vi "QueuedWriteToDatabase.vi"(8 "error in":errorcluster, 10 "Stop Flag Reference":refnum<vi>, 11 "queue":refnum<queue>) -> (0 "error out":errorcluster)   [LabVIEW 2014]
uses:
  <vilib>/addons/database/Connection.llb/Conn ObjectReference.ctl
  <vilib>/addons/database/NI_Database_API.lvlib
panel:
  out "Database Writing Source":i32
  out "Database Table":string
  out "Database Writing Error":bool
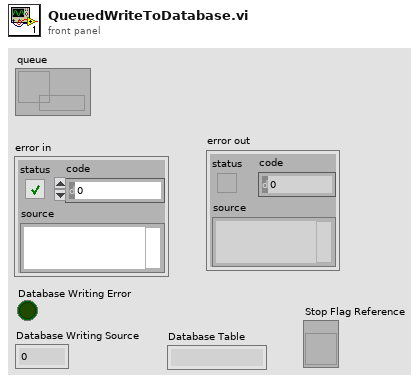
[diagram p1: front panel]
types:
  T1 = cluster{"setup":u8, "session_start_time":u64, "stim_start_time":u64, "time":u64}
  T2 = cluster{"setup":u8, "subject_id":i32, "session_start_time":dbl, "stim_start_time":dbl, "stim_path":path, "exp_type":string}
  T3 = cluster{"setup":u8, "subject_id":i32, "session_start_time":dbl, "stim_start_time":dbl, "time":dbl}
  T4 = cluster{"setup":u8, "subject_id":i32, "session_start_time":dbl, "stim_start_time":dbl, "beh_start_time":dbl, "beh_path":path, "beh_traces_type":string, "beh_stop_time":dbl}
  T5 = cluster{"setup":u8, "subject_id":i32, "session_start_time":dbl, "ephys_start_time":dbl, "ephys_path":path, "ephys_task":string, "ephys_stop_time":dbl}
  T6 = cluster{"setup":u8, "subject_id":u64, "session_start_time":dbl, "channel":u64, "counter":u64, "time":u64}
  T7 = cluster{"setup":u8, "subject_id":i32, "experimenter":string, "session_start_time":dbl, "session_path":path, "session_datetime":timestamp, "session_stop_time":dbl}
  T8 = cluster{"setup":u8, "subject_id":i32, "session_start_time":dbl, "stim_start_time":dbl, "stim_path":path, "exp_type":string, "stim_stop_time":dbl}
  T9 = typedef "NI_Database_API.lvlib/Conn ObjectReference.ctl" = refnum<k1>
  T10 = cluster{cluster{"reference":T9, "table":string, "columns":string[], i32}, "Variant":variant}
  T11 = cluster{"reference":T9, "table":string, "columns":string[], i32}
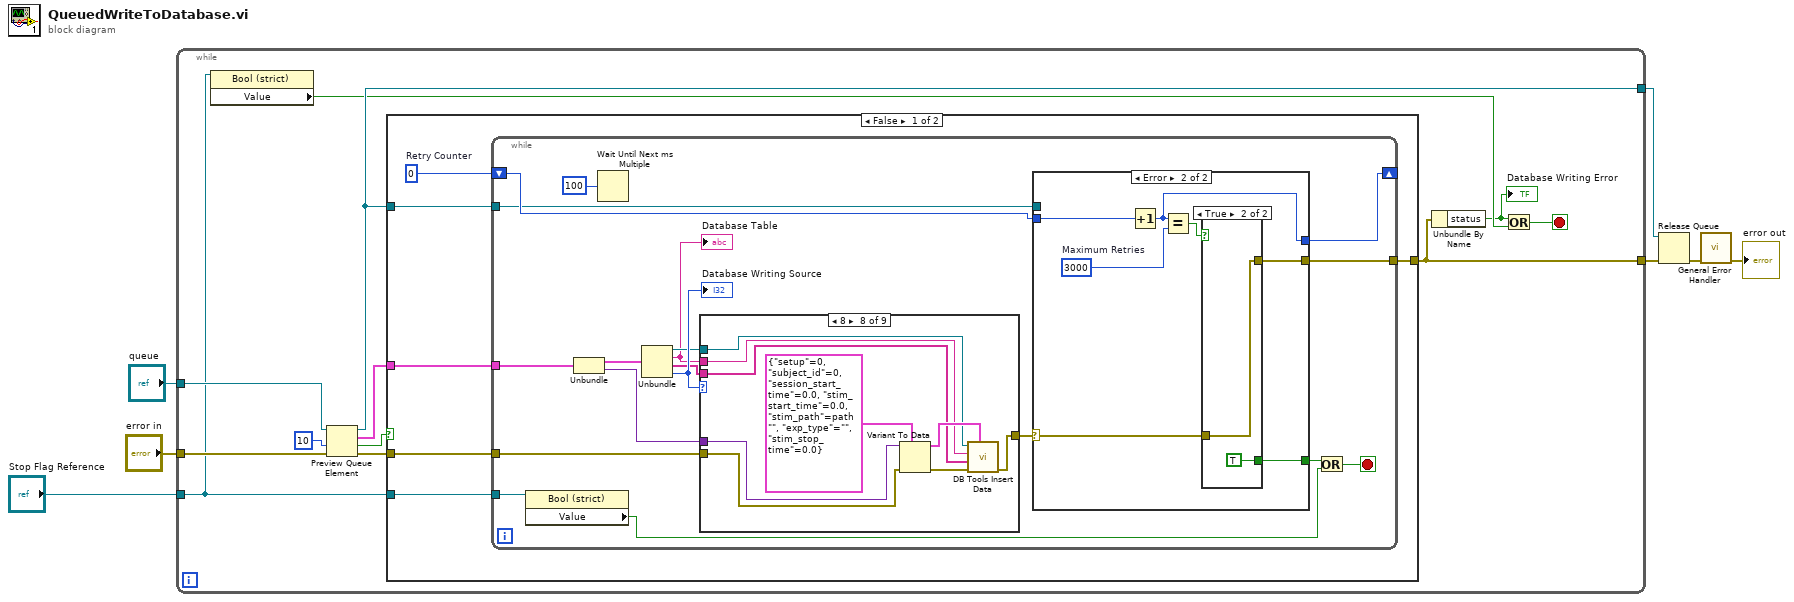
[diagram p0: block diagram]
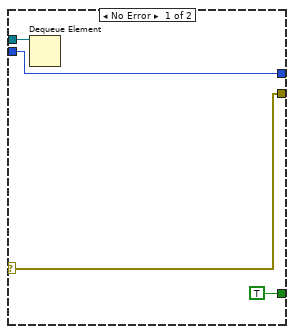
[diagram p2: hidden frame]
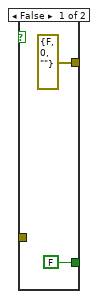
[diagram p3: hidden frame]
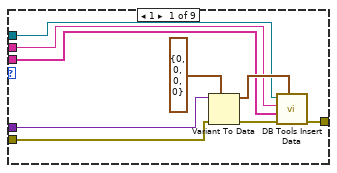
[diagram p4: hidden frame]
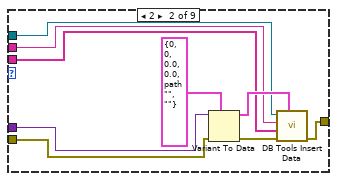
[diagram p5: hidden frame]
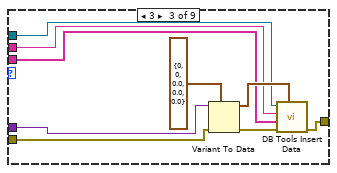
[diagram p6: hidden frame]
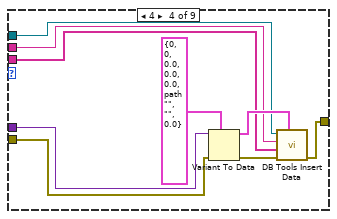
[diagram p7: hidden frame]
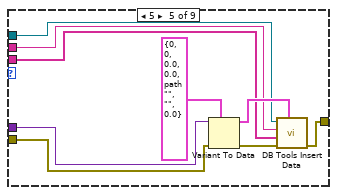
[diagram p8: hidden frame]
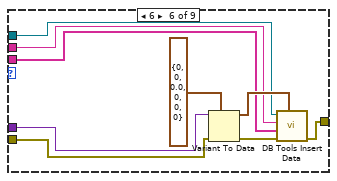
[diagram p9: hidden frame]
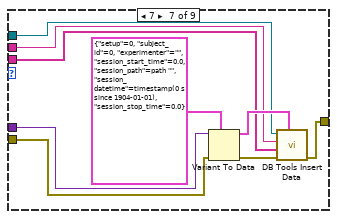
[diagram p10: hidden frame]
diagram:
  n1 = while {
    tunnel: "error in" -> [w13]
    tunnel: [w11] -> w4
    tunnel: [w12] -> w3
    tunnel: "Stop Flag Reference" -> [w8]
    tunnel: "queue" -> [w14]
    stop <- w16 stop-if-true
    n2 = property class="Bool (strict)"(reference=w8) -> ("Value"=w10:bool)  [unwired: 1 in, 2 out]
    n3 = Preview Queue Element(queue=w14, timeout in ms (-1)=10, error in (no error)=w13) -> (queue out=w11:refnum<queue>, element=w15:T10, timed out?=w18:bool, error out=w17:errorcluster)
    n4 = case shown="False" w18 {
      tunnel: w15 -> [w25 _]
      tunnel: w17 -> [w24 w132]
      tunnel: [w22 w132] -> w12
      tunnel: w11 -> [w21 _]
      tunnel: w8 -> [w20 _]
      frame False {
        w23 = 0  # Retry Counter
        n5 = while {
          tunnel: w25 -> [w43]
          tunnel: w24 -> [w39]
          shift-right: [w31] -> _
          shift-left: w23 -> [w33]
          tunnel: [w32] -> w22
          tunnel: w21 -> [w30]
          tunnel: w20 -> [w29]
          stop <- w27 stop-if-true
          n6 = property class="Bool (strict)"(reference=w29) -> ("Value"=w26:bool)  [unwired: 1 in, 2 out]
          n7 = Unbundle(w43) -> (w42:T11, "Variant"=w41:variant)
          n8 = Wait Until Next ms Multiple(millisecond multiple=u32 100) -> ()  [unwired: 1 out]
          n9 = Unbundle(w42) -> ("reference"=w38:T9, "table"=w37:string, "columns"=w36:string[], w40:i32)
          "Database Writing Source" <- w40
          "Database Table" <- w37
          n10 = case shown="8" w40 {
            tunnel: w41 -> [w67 w75 w84 w87 w98 w105 w116 w124 _]
            tunnel: w39 -> [w65 w74 w83 w88 w97 w107 w115 w125 w131]
            tunnel: [w59 w68 w77 w89 w96 w106 w114 w123 w131] -> w34
            tunnel: w38 -> [w63 w72 w81 w90 w99 w108 w119 w128 _]
            tunnel: w37 -> [w62 w71 w80 w91 w100 w109 w118 w127 _]
            tunnel: w36 -> [w61 w70 w79 w92 w101 w110 w117 w126 _]
            frame 1 {
              n11 = Variant To Data(error in=w65, type=T1 {"setup"=0, "session_start_time"=0, "stim_start_time"=0, "time"=0} ("output cluster"), Variant=w67) -> (data=w64:T1, error out=w60:errorcluster)
              n12 = call <vilib>:"DB Tools Insert Data.vi"("data"=w64, "error in (no error)"=w60, "columns"=w61, "table"=w62, "connection reference"=w63) -> ("error out"=w59:errorcluster)  [unwired: 5 in, 1 out]
            }
            frame 2 {
              n13 = Variant To Data(error in=w74, type=T2 {"setup"=0, "subject_id"=0, "session_start_time"=0.0, "stim_start_time"=0.0, "stim_path"=path "", "exp_type"=""} ("output cluster"), Variant=w75) -> (data=w73:T2, error out=w69:errorcluster)
              n14 = call <vilib>:"DB Tools Insert Data.vi"("data"=w73, "error in (no error)"=w69, "columns"=w70, "table"=w71, "connection reference"=w72) -> ("error out"=w68:errorcluster)  [unwired: 5 in, 1 out]
            }
            frame 3 {
              n15 = Variant To Data(error in=w83, type=T3 {"setup"=0, "subject_id"=0, "session_start_time"=0.0, "stim_start_time"=0.0, "time"=0.0} ("output cluster"), Variant=w84) -> (data=w82:T3, error out=w78:errorcluster)
              n16 = call <vilib>:"DB Tools Insert Data.vi"("data"=w82, "error in (no error)"=w78, "columns"=w79, "table"=w80, "connection reference"=w81) -> ("error out"=w77:errorcluster)  [unwired: 5 in, 1 out]
            }
            frame 4 {
              n17 = Variant To Data(error in=w88, type=T4 {"setup"=0, "subject_id"=0, "session_start_time"=0.0, "stim_start_time"=0.0, "beh_start_time"=0.0, "beh_path"=path "", "beh_traces_type"="", "beh_stop_time"=0.0} ("output cluster"), Variant=w87) -> (data=w93:T4, error out=w94:errorcluster)
              n18 = call <vilib>:"DB Tools Insert Data.vi"("data"=w93, "error in (no error)"=w94, "columns"=w92, "table"=w91, "connection reference"=w90) -> ("error out"=w89:errorcluster)  [unwired: 5 in, 1 out]
            }
            frame 5 {
              n19 = Variant To Data(error in=w97, type=T5 {"setup"=0, "subject_id"=0, "session_start_time"=0.0, "ephys_start_time"=0.0, "ephys_path"=path "", "ephys_task"="", "ephys_stop_time"=0.0} ("output cluster"), Variant=w98) -> (data=w102:T5, error out=w103:errorcluster)
              n20 = call <vilib>:"DB Tools Insert Data.vi"("data"=w102, "error in (no error)"=w103, "columns"=w101, "table"=w100, "connection reference"=w99) -> ("error out"=w96:errorcluster)  [unwired: 5 in, 1 out]
            }
            frame 6 {
              n21 = Variant To Data(error in=w107, type=T6 {"setup"=0, "subject_id"=0, "session_start_time"=0.0, "channel"=0, "counter"=0, "time"=0} ("output cluster"), Variant=w105) -> (data=w112:T6, error out=w111:errorcluster)
              n22 = call <vilib>:"DB Tools Insert Data.vi"("data"=w112, "error in (no error)"=w111, "columns"=w110, "table"=w109, "connection reference"=w108) -> ("error out"=w106:errorcluster)  [unwired: 5 in, 1 out]
            }
            frame 7 {
              n23 = Variant To Data(error in=w115, type=T7 {"setup"=0, "subject_id"=0, "experimenter"="", "session_start_time"=0.0, "session_path"=path "", "session_datetime"=timestamp(0 s since 1904-01-01), "session_stop_time"=0.0} ("output cluster"), Variant=w116) -> (data=w121:T7, error out=w120:errorcluster)
              n24 = call <vilib>:"DB Tools Insert Data.vi"("data"=w121, "error in (no error)"=w120, "columns"=w117, "table"=w118, "connection reference"=w119) -> ("error out"=w114:errorcluster)  [unwired: 5 in, 1 out]
            }
            frame 8 {
              n25 = Variant To Data(error in=w125, type=T8 {"setup"=0, "subject_id"=0, "session_start_time"=0.0, "stim_start_time"=0.0, "stim_path"=path "", "exp_type"="", "stim_stop_time"=0.0} ("Cluster"), Variant=w124) -> (data=w129:T8, error out=w130:errorcluster)
              n26 = call <vilib>:"DB Tools Insert Data.vi"("data"=w129, "error in (no error)"=w130, "columns"=w126, "table"=w127, "connection reference"=w128) -> ("error out"=w123:errorcluster)  [unwired: 5 in, 1 out]
            }
            frame 0, Default {
            }
          }
          n27 = case shown="Error" w34 {
            selector: w34 -> [w46 w50]
            tunnel: w33 -> [w47 w54]
            tunnel: [w47 w52] -> w31
            tunnel: [w46 w49] -> w32
            tunnel: [TRUE w48] -> w28
            tunnel: w30 -> [w44 _]
            frame No Error {
              n28 = Dequeue Element(queue=w44) -> ()  [unwired: 2 in, 4 out]
            }
            frame Error {
              w51 = 3000  # Maximum Retries
              n29 = Increment(x=w54) -> (x+1=w52:i32)
              n30 = Equal?(x=w52, y=w51) -> (x = y?=w53:bool)
              n31 = case shown="True" w53 {
                tunnel: w50 -> [_ w58]
                tunnel: [errorcluster {"status"=FALSE, "code"=0, "source"=""} ("error IO") w58] -> w49
                tunnel: [FALSE TRUE] -> w48
                frame False {
                }
                frame True {
                }
              }
            }
          }
          n32 = Or(x=w28, y=w26) -> (x .or. y?=w27:bool)
        }
      }
      frame True {
      }
    }
    n33 = Unbundle By Name(w12) -> ("status"=w9:bool)
    "Database Writing Error" <- w9
    n34 = Or(x=w9, y=w10) -> (x .or. y?=w16:bool)
  }
  n35 = Release Queue(queue=w4, error in (no error)=w3) -> (error out=w5:errorcluster)  [unwired: 1 in, 2 out]
  n36 = call <vilib>:"General Error Handler.vi"("error in (no error)"=w5) -> ("error out"=→"error out":errorcluster)  [unwired: 10 in, 4 out]
